vi "Parse XML Heap New.vi"(8 "error in (no error)":errorcluster, 11 "XML":string) -> (0 "error out":errorcluster, 3 "Items":refnum<class "Data Item.lvclass">[](array[class]))   [LabVIEW 2026, in "VILab.lvlib"]
uses:
  VILab.lvlib
  Classes/Data Item/Data Item.lvclass
  <vilib>/xml/Load XML String.vi
  <vilib>/xml/Close Reference(Node).vi
  <vilib>/xml/NI_XML.lvlib
  <resource>/objmgr/DOMUserDefRef.rc
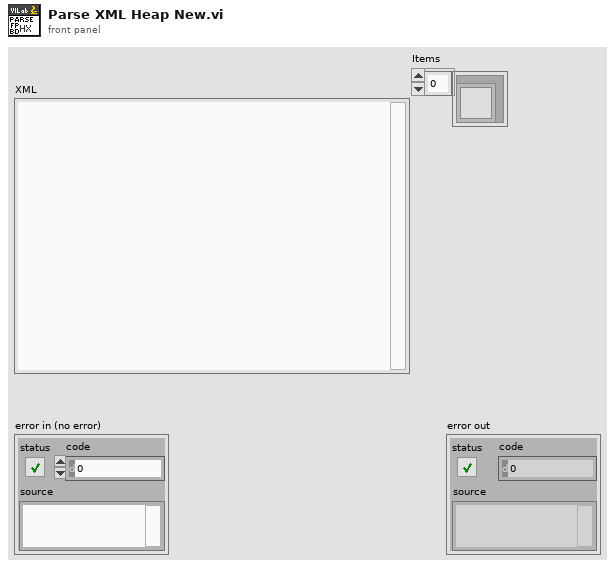
[diagram p1: front panel]
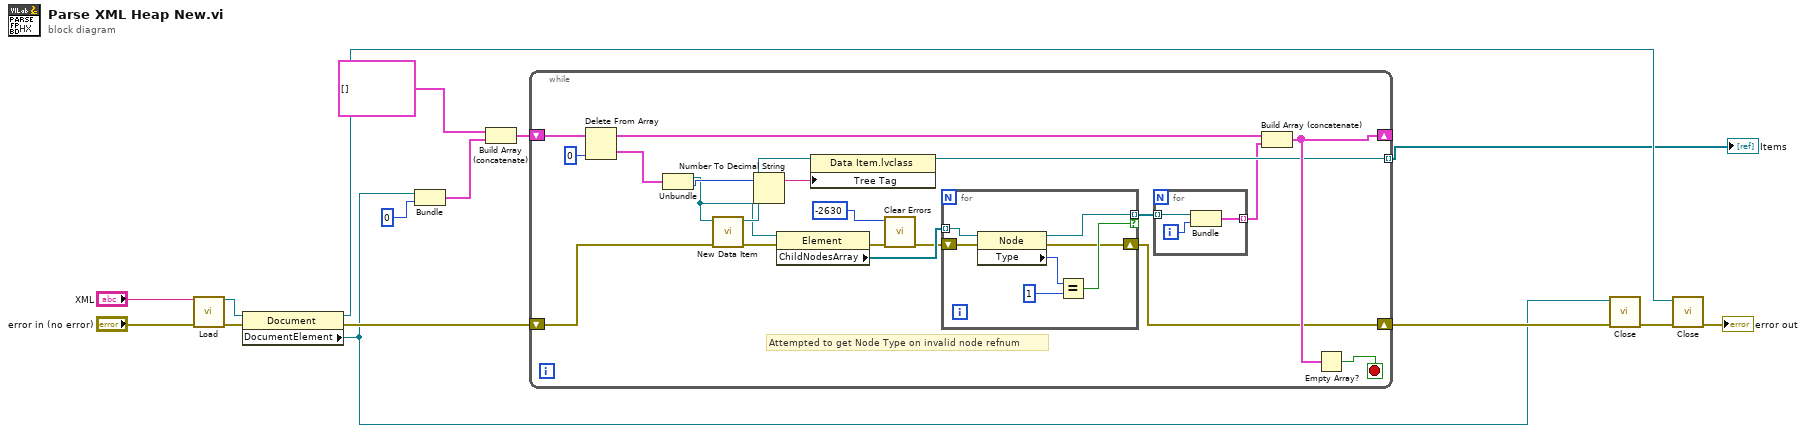
[diagram p0: block diagram]
diagram:
  n1 = call-poly <vilib>:"Load.vi"("XML string"="XML", "error in (no error)"="error in (no error)") -> ("DOM document out"=w8:refnum<k20>, "error out"=w15:errorcluster)  [unwired: 11 in, 1 out]
  n2 = property class="Document"(reference=w8, error in=w15) -> (reference out=w7:refnum<k20>, error out=w14:errorcluster, "DocumentElement"=w4:refnum<k20>)
  n3 = Bundle("DocumentElement"=w4, 0) -> (w2:cluster{"DocumentElement":refnum<k20>, i32})  [unwired: 1 in]
  n4 = Build Array (concatenate)(cluster{"Node":refnum<k20>, i32}[] [], w2) -> (w5:cluster{"DocumentElement":refnum<k20>, i32}[])
  n5 = while {
    shift-right: [w16] -> w12
    shift-left: w14 -> [w25]
    shift-right: [w32] -> _
    shift-left: w5 -> [w35]
    tunnel: [w20] -> w1 mode=indexing
    stop <- w31 stop-if-true
    # "Attempted to get Node Type on invalid node refnum"
    n6 = Delete From Array(array=w35, index=0) -> (deleted portion=w24:cluster{"DocumentElement":refnum<k20>, i32}, array with subset deleted=w34:cluster{"DocumentElement":refnum<k20>, i32}[])  [unwired: 1 in]
    n7 = Unbundle(w24) -> ("DocumentElement"=w17:refnum<k20>, w21:i32)
    n8 = call "New Data Item.vi"("error in (no error)"=w25, "node in"=w17) -> ("error out"=w27:errorcluster, "Data Item"=w23:refnum<class "Data Item.lvclass">)  [unwired: 8 in]
    n9 = Number To Decimal String(number=w21) -> (decimal integer string=w22:string)  [unwired: 1 in]
    n10 = property class="Element"(reference=w17, error in=w27) -> (error out=w29:errorcluster, "ChildNodesArray"=w30:refnum<k20>[])  [unwired: 1 out]
    n11 = property class="Data Item.lvclass"(reference=w23, "Tree Tag"=w22) -> (reference out=w20:refnum<class "Data Item.lvclass">)  [unwired: 1 in, 1 out]
    n12 = call <vilib>:"Clear Errors.vi"("error in (no error)"=w29, "specific error code to clear (0: all)"=-2630) -> ("error out"=w28:errorcluster)  [unwired: 4 in, 1 out]
    n13 = for {
      shift-right: [w39] -> w16
      shift-left: w28 -> [w45]
      tunnel: w30 -> [w44] mode=indexing
      tunnel: [w41] -> w19 mode=indexing if=w40
      n14 = property class="Node"(reference=w44, error in=w45) -> (reference out=w41:refnum<k20>, error out=w39:errorcluster, "Type"=w43:i32)
      n15 = Equal?(x=w43, y=1) -> (x = y?=w40:bool)
    }
    n16 = for {
      tunnel: w19 -> [w38] mode=indexing
      tunnel: [w36] -> w18 mode=indexing
      i -> [w37]
      n17 = Bundle(w38, w37) -> (w36:cluster{refnum<k20>, i32})  [unwired: 1 in]
    }
    n18 = Build Array (concatenate)(w34, w18) -> (w32:cluster{"DocumentElement":refnum<k20>, i32}[])
    n19 = Empty Array?(array=w32) -> (empty?=w31:bool)
  }
  "Items" <- w1
  n20 = call-poly <vilib>:"Close.vi"("error in (no error)"=w12, "node"=w4) -> ("error out"=w13:errorcluster)  [unwired: 7 in]
  n21 = call-poly <vilib>:"Close.vi"("error in (no error)"=w13, "node"=w7) -> ("error out"=→"error out":errorcluster)  [unwired: 7 in]
